vi "LabViewTutorial4.vi"() -> ()   [LabVIEW 2014]
uses:
  <vilib>/express/express analysis/Spectral/Block/exnSpectralBlock spectral measurements peak poly.vi
  <vilib>/express/express analysis/Spectral/Block/exnSpectralBlock spectral measurements peak DDT.vi
  <vilib>/express/express analysis/Spectral/XNode/ExpressSpectralMeasurementsBlockNode.xnode
panel:
  in  "Standard deviation":dbl=0.6
  in  "Slide":dbl(slide) scale=0.0..2.0
  out "Frequency":dbl
  out "Amplitude":dbl
  in  "Amplitude":dbl(knob)=1.0 scale=0.0..10.0
  in  "Frequency":dbl(knob)=10.1 scale=0.0..250.0
  in  "Offset":dbl(knob) scale=0.0..10.0
  in  "stop":bool
  in  "Tab Control":enum32{"AFG", "FFT"}(tab)
  out "Sine":dynamicdata(graph)
  out "Waveform Graph":dynamicdata(graph)
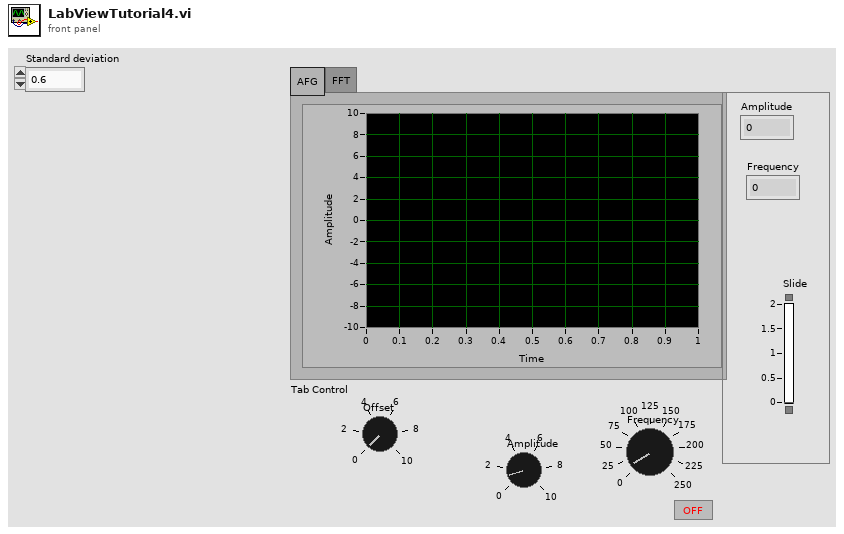
[diagram p1: front panel]
types:
  T1 = cluster{"averaging mode":u16, "weighting mode":u16, "number of averages":u32}
  T2 = cluster{"dB On (F)":bool, "unwrap phase (F)":bool, "convert to degree (F)":bool}
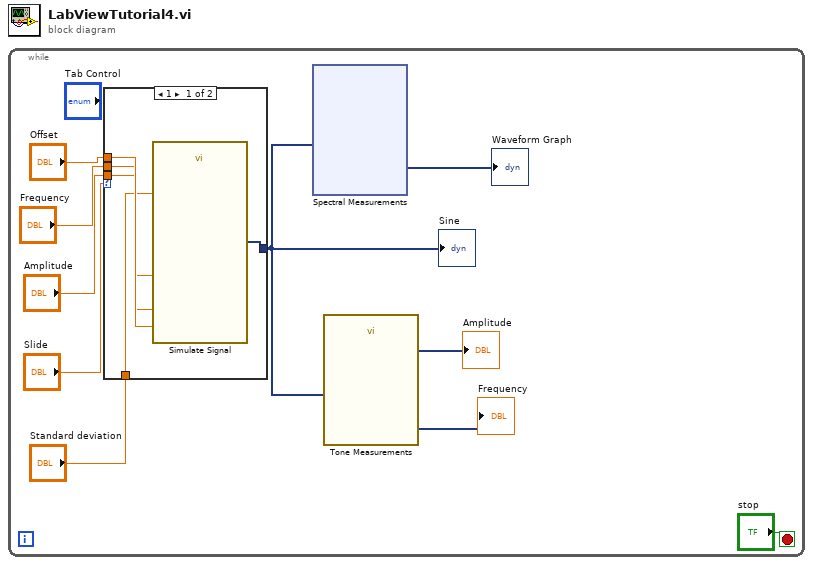
[diagram p0: block diagram]
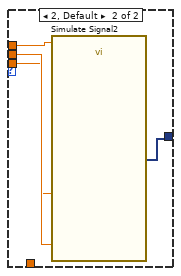
[diagram p2: hidden frame]
diagram:
  n1 = while {
    stop <- "stop" stop-if-true
    n2 = case shown="1" "Slide" {
      tunnel: "Offset" -> [w15 w18]
      tunnel: "Frequency" -> [w14 w17]
      tunnel: "Amplitude" -> [w13 w16]
      tunnel: [w12 w19] -> w6
      tunnel: "Standard deviation" -> [w11 _]
      frame 1 {
        n3 = call "Simulate Signal"("Offset"=w15, "Frequency"=w14, "Amplitude"=w13, "Standard deviation"=w11) -> ("Sine with Gaussian Noise"=w12:dynamicdata)  [unwired: 10 in, 1 out]
      }
      frame 2, Default {
        n4 = call "Simulate Signal2"("Offset"=w18, "Frequency"=w17, "Amplitude"=w16) -> ("Square with Uniform Noise"=w19:dynamicdata)  [unwired: 11 in, 1 out]
      }
    }
    "Sine" <- w6
    n5 = xnode "Spectral Measurements"("Signals"=w6) -> ("FFT - (Peak)"=→"Waveform Graph":dynamicdata)  [unwired: 1 in, 2 out]
    n6 = call "Tone Measurements"("Signals"=w6) -> ("Frequency"=→"Frequency":dynamicdata, "Amplitude"=→"Amplitude":dynamicdata)  [unwired: 8 in, 1 out]
  }
